vi "Format-shooter-speed-mode.vi"() -> (1 "Shooter Speed Mode Color":u32, 3 "Shooter Speed Mode Text":string)   [LabVIEW 2020]
uses:
  <vilib>/Rock Robotics/Network Tables/NT Read Number.vi
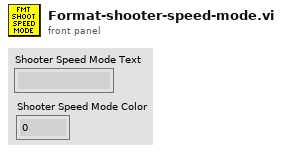
[diagram p1: front panel]
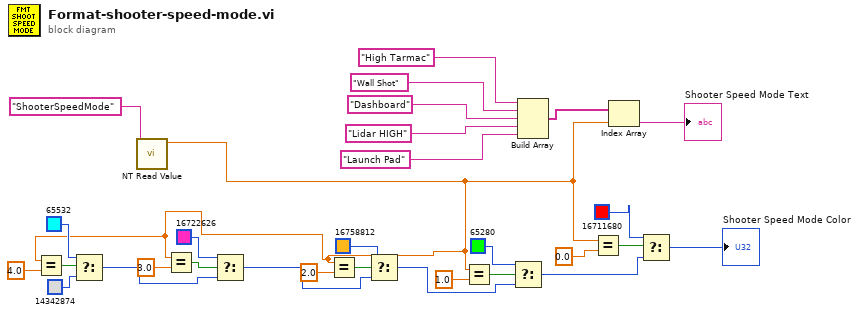
[diagram p0: block diagram]
diagram:
  n1 = call-poly <vilib>:"NT Read Value.vi"("name"="ShooterSpeedMode" ("Name")) -> ("value"=w26:dbl)  [unwired: 8 in, 2 out]
  n2 = Equal?(x=w26, y=4.0) -> (x = y?=w25:bool)
  n3 = Select(t=u32 65532 ("Text.Colors:BG Color"), s=w25, f=u32 14342874 ("Text.Colors:BG Color")) -> (s? t:f=w24:u32)
  n4 = Equal?(x=w26, y=3.0) -> (x = y?=w21:bool)
  n5 = Select(t=u32 16722626 ("Text.Colors:BG Color"), s=w21, f=w24) -> (s? t:f=w20:u32)
  n6 = Equal?(x=w26, y=2.0) -> (x = y?=w18:bool)
  n7 = Select(t=u32 16758812 ("Text.Colors:BG Color"), s=w18, f=w20) -> (s? t:f=w16:u32)
  n8 = Equal?(x=w26, y=1.0) -> (x = y?=w14:bool)
  n9 = Select(t=u32 65280 ("Text.Colors:BG Color"), s=w14, f=w16) -> (s? t:f=w12:u32)
  n10 = Build Array("High Tarmac", "Wall Shot", "Dashboard", "Lidar HIGH", "Launch Pad") -> (w9:string[])
  n11 = Equal?(x=w26, y=0.0) -> (x = y?=w10:bool)
  n12 = Index Array(array=w9, index=w26) -> (element=→"Shooter Speed Mode Text":string)
  n13 = Select(t=u32 16711680 ("Text.Colors:BG Color"), s=w10, f=w12) -> (s? t:f=→"Shooter Speed Mode Color":u32)
